vi "selevt indicators.vi"(10 "Zone Selector":T1, 11 "sprinkler data in":T2 {"Zone Indicators"."Timing" format="%#.2g"}) -> (3 "sprinkler data out":T2 {"Zone Indicators"."Timing" format="%#.2g"})   [LabVIEW 2015]
uses:
  controls/sprinkler data.ctl
  Solution/Controls/Zone Setup.ctl
  Solution/Controls/Zone.ctl
  Solution/Controls/Zone Indicators.ctl
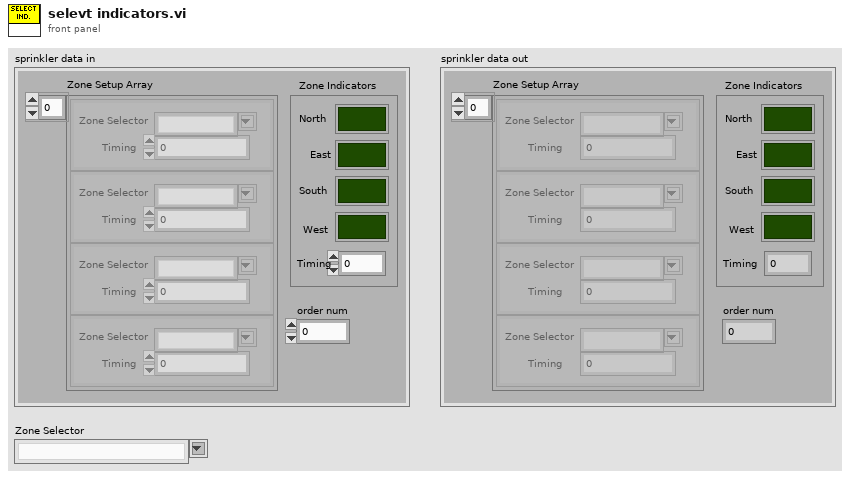
[diagram p1: front panel]
types:
  T1 = typedef "Zone.ctl" = string
  T2 = typedef "sprinkler data.ctl" = cluster{"Zone Setup Array":T3[], "Zone Indicators":T4, "order num":i32}
  T3 = typedef "Zone Setup.ctl" = cluster{"Zone Selector":T1, "Timing":u32}
  T4 = typedef "Zone Indicators.ctl" = cluster{"North":bool, "East":bool, "South":bool, "West":bool, "Timing":dbl}
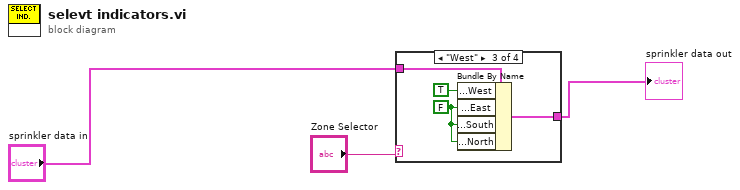
[diagram p0: block diagram]
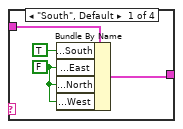
[diagram p2: hidden frame]
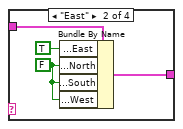
[diagram p3: hidden frame]
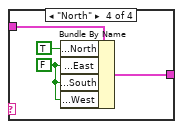
[diagram p4: hidden frame]
diagram:
  n1 = case shown="\"West\"" "Zone Selector" {
    tunnel: "sprinkler data in" -> [w6 w11 w15 w19]
    tunnel: [w7 w10 w12 w16] -> w3
    frame "South", Default {
      w4 = FALSE ("Zone Indicators.East")
      n2 = Bundle By Name(cluster=w6, "Zone Indicators.South"=TRUE, "Zone Indicators.East"=w4, "Zone Indicators.North"=w4, "Zone Indicators.West"=w4) -> (w7:T2)
    }
    frame "East" {
      w8 = FALSE ("Zone Indicators.North")
      n3 = Bundle By Name(cluster=w11, "Zone Indicators.East"=TRUE, "Zone Indicators.North"=w8, "Zone Indicators.South"=w8, "Zone Indicators.West"=w8) -> (w10:T2)
    }
    frame "West" {
      w13 = FALSE ("Zone Indicators.East")
      n4 = Bundle By Name(cluster=w15, "Zone Indicators.West"=TRUE, "Zone Indicators.East"=w13, "Zone Indicators.South"=w13, "Zone Indicators.North"=w13) -> (w12:T2)
    }
    frame "North" {
      w17 = FALSE ("Zone Indicators.East")
      n5 = Bundle By Name(cluster=w19, "Zone Indicators.North"=TRUE, "Zone Indicators.East"=w17, "Zone Indicators.South"=w17, "Zone Indicators.West"=w17) -> (w16:T2)
    }
  }
  "sprinkler data out" <- w3
